vi "CAN_Init.vi"(0 "object in":refnum<class "CAN.lvclass">, 5 "Init Data":T1={"XNET Interface"="", "Baud Rate"=500000, "CAN:Termination"=0, "Echo Transmit?"=FALSE, "scope (normal)"=1} {"scope (normal)" items=["Normal", "Session Only", "Interface Only", "Session Only Blocking"]; "CAN:Termination" items=["Off", "On"]; "Baud Rate" format="%.0p"}, 11 "error in (no error)":errorcluster) -> (4 "object out":refnum<class "CAN.lvclass">, 15 "error out":errorcluster)   [LabVIEW 2023, in "HardwareAbstractionLayer_LVOOP.lvlib" / "CAN HAL Lib.lvlib" / "CAN.lvclass"]
uses:
  CAN.lvclass
  Ctrls/CAN Init Ctrl.ctl
  <vilib>/xnet/xnet.llb/XNET Control Scope.ctl
  CAN.lvclass/CAN.ctl
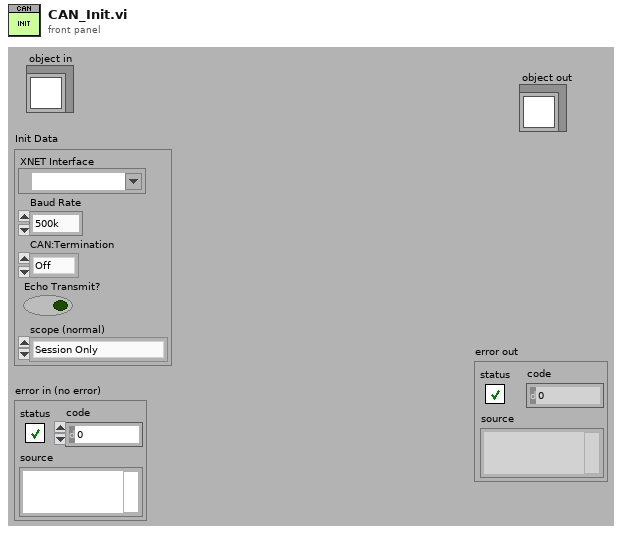
[diagram p1: front panel]
types:
  T1 = typedef "HardwareAbstractionLayer_LVOOP.lvlib/CAN HAL Lib.lvlib/CAN.lvclass/CAN Init Ctrl.ctl" = cluster{"XNET Interface":refnum<k21>, "Baud Rate":u64, "CAN:Termination":u32, "Echo Transmit?":bool, "scope (normal)":T2}
  T2 = typedef "XNET Control Scope.ctl" = u32
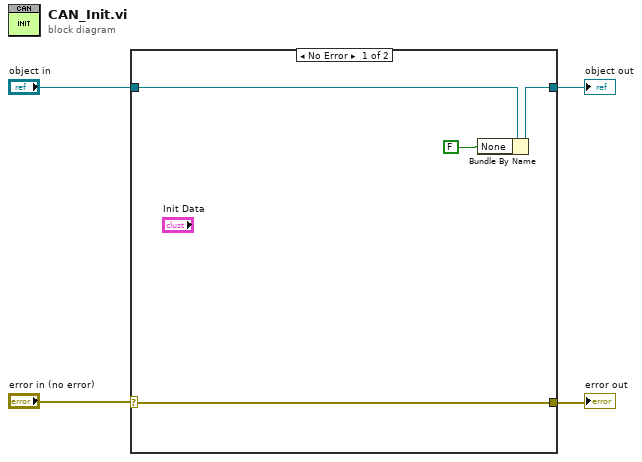
[diagram p0: block diagram]
diagram:
  n1 = case shown="No Error" "error in (no error)" {
    selector: "error in (no error)" -> [w5 w9]
    tunnel: "object in" -> [w8 w10]
    tunnel: [w7 w10] -> w3
    tunnel: [w5 w9] -> w1
    frame No Error {
      n2 = Bundle By Name(cluster=w8, "None"=FALSE) -> (w7:refnum<class "CAN.lvclass">)
    }
    frame Error {
    }
  }
  "object out" <- w3
  "error out" <- w1
